vi "HEWH Full Cutout Check.vi"(7 "Station Data Input":T1={"Sequence #"=0.0, "Cycles"=0, "Mode Setting"="", "Flow Rate (GPM)"=0.0, "Temperature (F)"=0.0, "Reset Timer"=FALSE, "Use Temp Decline Method"=FALSE, "Terminate Condition"=enum."C1-Terminate Draw @ Gallon Mark", "Condition Value #1"=0.0, "UE"=FALSE, "LE"=FALSE, "Comp"=FALSE, "Fan"=FALSE, "Test End Time (Sec)"=0.0, "Purge Until Cutout"=FALSE, "Start Conditions"=enum."Heat Source Cutout", "Condition Value #2"=0.0, "Remove Power"=FALSE, "Time"=0.0, "Check Special Cond."=enum."SC2-Check Heat Source (On-C2/Off-C1)", "Condition#"=enum."C1", "Draw Flags"=enum."N/A", "Data Processing Delay (FHD 15sec, UEF 5 Sec)"=0.0, "Test Complete"=FALSE} {"Time" format="%<%H:%M:%S>t"}, 8 "Error In":errorcluster, 11 "POWER":T8) -> (0 "Error Out":errorcluster, 3 "Heat Source ON (1=ON)":bool, 5 "Skip Current Check":bool)   [LabVIEW 2016]
uses:
  Type Definitions/HEWH Power Elements.ctl
  Type Definitions/PRAT Test.ctl
  Utility/Save File/File Setup (Public)/Type Definition/Save File HEWH Heating Control Mode.ctl
  Draw Water Specific/Type Definitions/Terminate Draw Conditions.ctl
  Type Definitions/HEWH Start Conditions.ctl
  Draw Water Specific/Type Definitions/Check Special Condtions.ctl
  Draw Water Specific/Type Definitions/HEWH Special Condition Check.ctl
  Type Definitions/HEWH Draw Flag ENUM.ctl
  Utility/Save File/File Setup.lvlib
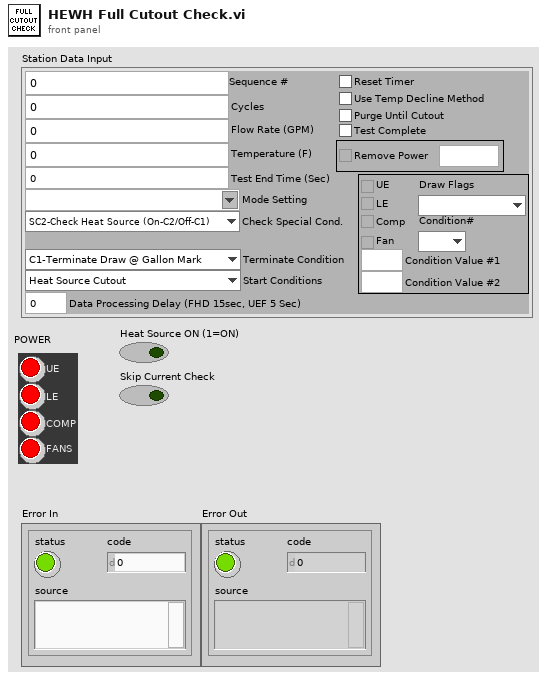
[diagram p1: front panel]
types:
  T1 = typedef "PRAT Test.ctl" = cluster{"Sequence #":dbl, "Cycles":i32, "Mode Setting":T2, "Flow Rate (GPM)":dbl, "Temperature (F)":dbl, "Reset Timer":bool, "Use Temp Decline Method":bool, "Terminate Condition":T3, "Condition Value #1":dbl, "UE":bool, "LE":bool, "Comp":bool, "Fan":bool, "Test End Time (Sec)":dbl, "Purge Until Cutout":bool, "Start Conditions":T4, "Condition Value #2":dbl, "Remove Power":bool, "Time":dbl, "Check Special Cond.":T5, "Condition#":T6, "Draw Flags":T7, "Data Processing Delay (FHD 15sec, UEF 5 Sec)":dbl, "Test Complete":bool}
  T2 = typedef "File Setup.lvlib/Save File HEWH Heating Control Mode.ctl" = string
  T3 = typedef "Terminate Draw Conditions.ctl" = enum16{"C1-Terminate Draw @ Gallon Mark", "C2-Special Last Draw (HU Test)", "C3-RTD Out <=", "C4-Mean Tank Temp <=", "C5-Decrease RTD Out (Deg F)", "C6-Time (Seconds)", "C7-Until Any Heat Source", "C8-Specific Heat Source", "C9-Do Nothing"}
  T4 = typedef "HEWH Start Conditions.ctl" = enum16{"Heat Source Cutout", "At Time (Seconds)", "Every X (Seconds)", "T2 >= X° Below Setpoint", "Seconds From Complete", "Wait for LE & Comp Cutout", "Wait for Comp Cutout", "Wait for LE Cutout", "Wait for UE Cutout"}
  T5 = typedef "Check Special Condtions.ctl" = enum16{"SC1-Do Nothing", "SC2-Check Heat Source (On-C2/Off-C1)", "SC3-Check Skip Condition", "SC4-Check Heat Source ON/Fail"}
  T6 = typedef "HEWH Special Condition Check.ctl" = enum16{"N/A", "C1", "C2", "Reset/Fail", "Skip Draw Sequence"}
  T7 = typedef "HEWH Draw Flag ENUM.ctl" = enum16{"N/A", "None(0)", "Sml(1)", "Med(2)", "SmlMed(3)", "Lrg(4)", "SmlLrg(5)", "MedLrg(6)", "SmlMedLrg(7)"}
  T8 = typedef "HEWH Power Elements.ctl" = cluster{"UE":bool, "LE":bool, "COMP":bool, "FANS":bool}
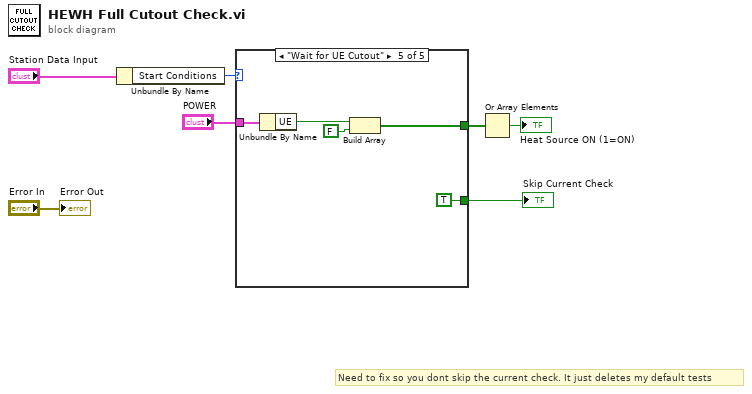
[diagram p0: block diagram]
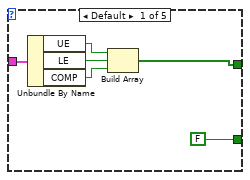
[diagram p2: hidden frame]
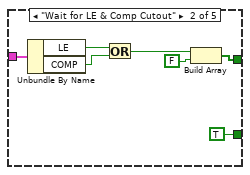
[diagram p3: hidden frame]
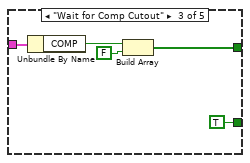
[diagram p4: hidden frame]
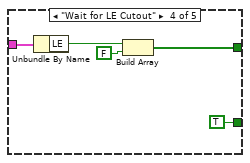
[diagram p5: hidden frame]
diagram:
  # "Need to fix so you dont skip the current check. It just deletes my default tests"
  n1 = Unbundle By Name("Station Data Input") -> ("Start Conditions"=w3:T4)
  n2 = case shown="\"Wait for UE Cutout\"" w3 {
    tunnel: [w12 w17 w22 w27 w32] -> w6
    tunnel: "POWER" -> [w10 w20 w25 w30 w33]
    tunnel: [FALSE ("logical OR") TRUE ("logical OR") TRUE ("logical OR") TRUE ("logical OR") TRUE ("logical OR")] -> w1
    frame Default {
      n3 = Unbundle By Name(w10) -> ("UE"=w9:bool, "LE"=w11:bool, "COMP"=w13:bool)
      n4 = Build Array(w9, w11, w13) -> (w12:bool[])
    }
    frame "Wait for LE & Comp Cutout" {
      n5 = Unbundle By Name(w20) -> ("LE"=w16:bool, "COMP"=w15:bool)
      n6 = Or(x=w16, y=w15) -> (x .or. y?=w19:bool)
      n7 = Build Array(w19, FALSE ("element")) -> (w17:bool[])
    }
    frame "Wait for Comp Cutout" {
      n8 = Unbundle By Name(w25) -> ("COMP"=w24:bool)
      n9 = Build Array(w24, FALSE ("element")) -> (w22:bool[])
    }
    frame "Wait for LE Cutout" {
      n10 = Unbundle By Name(w30) -> ("LE"=w29:bool)
      n11 = Build Array(w29, FALSE ("element")) -> (w27:bool[])
    }
    frame "Wait for UE Cutout" {
      n12 = Unbundle By Name(w33) -> ("UE"=w35:bool)
      n13 = Build Array(w35, FALSE ("element")) -> (w32:bool[])
    }
  }
  "Skip Current Check" <- w1
  n14 = Or Array Elements(Boolean array=w6) -> (logical OR=→"Heat Source ON (1=ON)":bool)
  "Error Out" <- "Error In"
